vi "estiUk.vi"(5 "y2 Matrix":dbl[][](array[numeric]), 6 "Optical State":dbl[](array[numeric]), 7 "Sen M":dbl[][][](array[numeric]), 8 "error in (no error)":errorcluster, 9 "Effective Wavelength":dbl, 10 "Idx Group":cluster{"zn3Idx":i32[], "dofIdx":i32[]}, 11 "OptCtrl in":refnum<class "OptCtrl.lvclass">) -> (0 "error out":errorcluster, 2 "uk Array":dbl[](array[numeric]), 3 "OptCtrl out":refnum<class "OptCtrl.lvclass">)   [LabVIEW 2016, in "OfcFunc.lvlib" / "OptCtrl.lvclass"]
doc: "Estimate uk by referencing to \"0\", \"x0\", or \"x00\" based on the configuration file."
uses:
  OptCtrl.lvclass
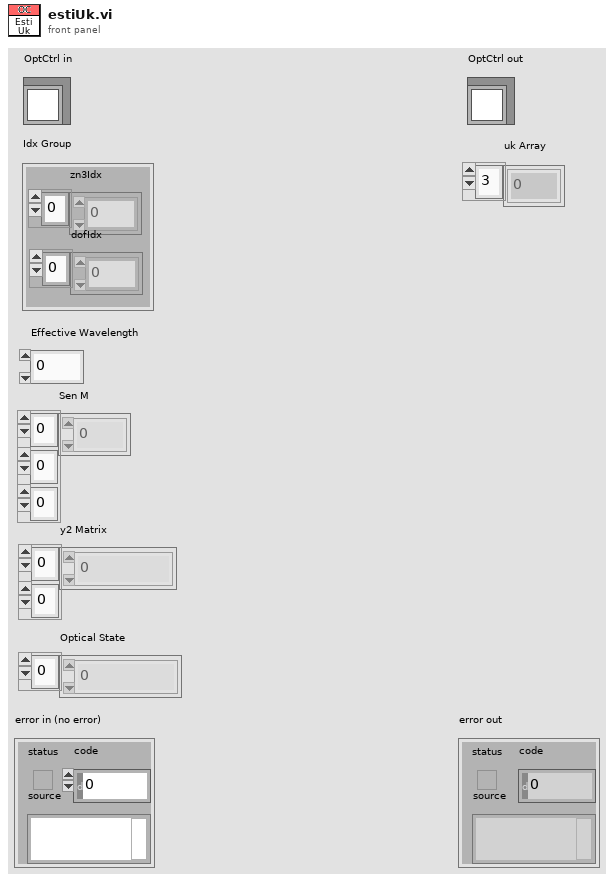
[diagram p1: front panel]
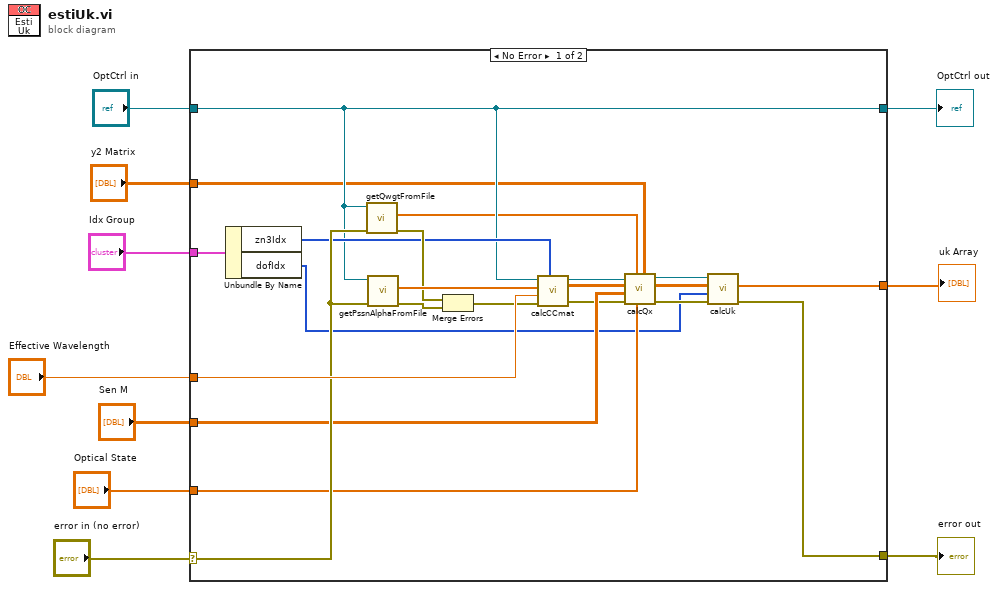
[diagram p0: block diagram]
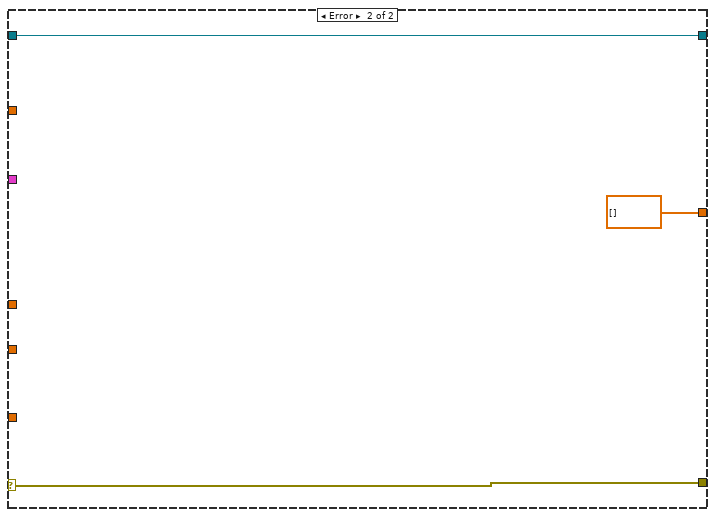
[diagram p2: hidden frame]
diagram:
  n1 = case shown="No Error" "error in (no error)" {
    selector: "error in (no error)" -> [w30 w35]
    tunnel: [w11 w35] -> w9
    tunnel: [w24 w34] -> w7
    tunnel: "OptCtrl in" -> [w24 w34]
    tunnel: "Effective Wavelength" -> [w31 _]
    tunnel: "Sen M" -> [w20 _]
    tunnel: "Idx Group" -> [w26 _]
    tunnel: "y2 Matrix" -> [w18 _]
    tunnel: "Optical State" -> [w17 _]
    tunnel: [w12 dbl[] [] ("uk Array")] -> w1
    frame No Error {
      n2 = Unbundle By Name(w26) -> ("zn3Idx"=w25:i32[], "dofIdx"=w13:i32[])
      n3 = call "getQwgtFromFile.vi"("error in (no error)"=w30, "OptCtrl in"=w24) -> ("error out"=w29:errorcluster, "Wgt of Q"=w22:dbl[])  [unwired: 7 in, 1 out]
      n4 = call "getPssnAlphaFromFile.vi"("error in (no error)"=w30, "OptCtrl in"=w24) -> ("error out"=w28:errorcluster, "PSSN Alpha"=w32:dbl[])  [unwired: 7 in, 1 out]
      n5 = Merge Errors(w29, w28) -> (w27:errorcluster)
      n6 = call "calcCCmat.vi"("zn3Idx"=w25, "error in (no error)"=w27, "Effective Wavelength"=w31, "PSSN Alpha"=w32, "OptCtrl in"=w24) -> ("error out"=w19:errorcluster, "CC Matrix"=w21:dbl[][], "OptCtrl out"=w23:refnum<class "OptCtrl.lvclass">)  [unwired: 4 in]
      n7 = call "calcQx.vi"("y2 Matrix"=w18, "Optical State"=w17, "Weighting of Field Point"=w22, "error in (no error)"=w19, "Sen M"=w20, "CC Matrix"=w21, "OptCtrl in"=w23) -> ("error out"=w14:errorcluster, "Qx Array"=w15:dbl[][], "OptCtrl out"=w16:refnum<class "OptCtrl.lvclass">)  [unwired: 2 in]
      n8 = call "calcUk.vi"("error in (no error)"=w14, "dofIdx"=w13, "Qx Array"=w15, "OptCtrl in"=w16) -> ("error out"=w11:errorcluster, "uk Array"=w12:dbl[])  [unwired: 5 in, 1 out]
    }
    frame Error {
    }
  }
  "error out" <- w9
  "OptCtrl out" <- w7
  "uk Array" <- w1
